vi "http_message_body.vi"(10 "String":string, 11 "HTTP Client in":T1) -> (2 "Boolean":bool, 3 "HTTP Client out":T1)   [LabVIEW 2011]
uses:
  tcp_client.ctl
  <vilib>/regexp/Match Regular Expression.xnode
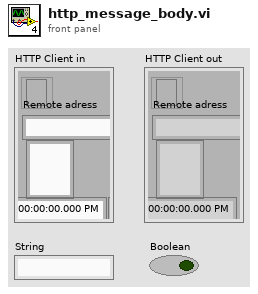
[diagram p1: front panel]
types:
  T1 = typedef "tcp_client.ctl" = cluster{"connection ID":refnum<k5>, "Buffer":string, "Remote adress":string, "accessed last time at":timestamp}
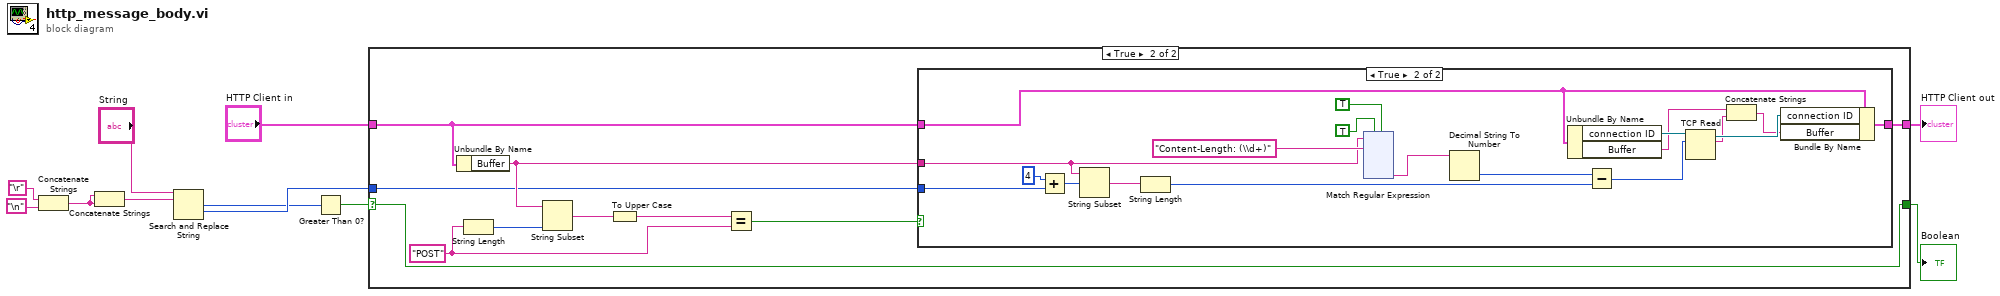
[diagram p0: block diagram]
diagram:
  n1 = Concatenate Strings("\r", "\n") -> (w7:string)
  n2 = Concatenate Strings(w7, w7) -> (w8:string)
  n3 = Search and Replace String(input string="String", search string=w8) -> (number of replacements=w9:i32, offset past replacement=w11:i32)  [unwired: 6 in, 2 out]
  n4 = Greater Than 0?(x=w9) -> (x > 0?=w10:bool)
  n5 = case shown="True" w10 {
    selector: w10 -> [w13 w23]
    tunnel: [w13 w23] -> w1
    tunnel: "HTTP Client in" -> [w12 w17]
    tunnel: [w12 w18] -> w3
    tunnel: w11 -> [_ w15]
    frame False {
    }
    frame True {
      w19 = "POST"
      n6 = Unbundle By Name(w17) -> ("Buffer"=w16:string)
      n7 = String Length(string=w19) -> (length=w22:i32)
      n8 = String Subset(string=w16, length (rest)=w22) -> (substring=w21:string)  [unwired: 1 in]
      n9 = To Upper Case(1:w21) -> (0:w20:string)
      n10 = Equal?(x=w20, y=w19) -> (x = y?=w14:bool)
      n11 = case shown="True" w14 {
        tunnel: [w24 w37] -> w18
        tunnel: w17 -> [w24 w39]
        tunnel: w16 -> [_ w33]
        tunnel: w15 -> [_ w32]
        frame False {
        }
        frame True {
          n12 = Add(x=4, y=w32) -> (x+y=w26:i32)
          n13 = String Subset(string=w33, offset (0)=w26) -> (substring=w31:string)  [unwired: 1 in]
          n14 = String Length(string=w31) -> (length=w30:i32)
          n15 = xnode "Match Regular Expression"("input string"=w33, "regular expression"="Content-Length: (\\d+)", "ignore case? (F)"=TRUE, "multiline? (F)"=TRUE) -> ("submatch 1"=w40:string)  [unwired: 2 in, 5 out]
          n16 = Decimal String To Number(string=w40) -> (number=w29:i32)  [unwired: 2 in, 1 out]
          n17 = Unbundle By Name(w39) -> ("connection ID"=w38:refnum<k5>, "Buffer"=w35:string)
          n18 = Subtract(x=w29, y=w30) -> (x-y=w28:i32)
          n19 = TCP Read(connection ID=w38, bytes to read=w28) -> (connection ID out=w36:refnum<k5>, data out=w34:string)  [unwired: 3 in, 1 out]
          n20 = Concatenate Strings(w35, w34) -> (w27:string)
          n21 = Bundle By Name(cluster=w39, "connection ID"=w36, "Buffer"=w27) -> (w37:T1)
        }
      }
    }
  }
  "HTTP Client out" <- w3
  "Boolean" <- w1
